vi "4channel.vi"() -> ()   [LabVIEW 2014]
doc: "Personal Daq 54 example.\nTriggering is immediate and readings are returned 1 scan at a time as available.\nBe sure to use the Acquisition Stop control for proper shutdown."
uses:
  <vilib>/Utility/error.llb/DialogType.ctl
  <vilib>/DAQmx/read.llb/DAQmx Read (Analog 1D DBL NChan 1Samp).vi
  <vilib>/Analysis/2dsp.llb/Complex FFT.vi
  <vilib>/DAQmx/create/channels.llb/DAQmx Create Channel (AI-Voltage-Basic).vi
  <vilib>/DAQmx/configure/timing.llb/DAQmx Timing (Sample Clock).vi
  <vilib>/DAQmx/miscellaneous.llb/DAQmx Fill In Error Info.vi
  <vilib>/measure/madcrms.llb/Basic Averaged DC-RMS for 1 Chan.vi
  Instance           2 26Saved   noise_Nov07_2009_5 .vi
  Instance          18 26Saved   noise_Nov07_2009_5 .vi
  <vilib>/express/express analysis/Spectral/Block/exnSpectralBlock spectral measurements peak poly.vi
  <vilib>/express/express analysis/Spectral/Block/exnSpectralBlock spectral measurements peak DDT.vi
  Instance           1 26Saved   noise_Nov07_2009_5 .vi
  Instance           4 26Saved   noise_Nov07_2009_5 .vi
  <vilib>/express/express analysis/Spectral/XNode/ExpressSpectralMeasurementsBlockNode.xnode
  <vilib>/measure/NI_MAPro.lvlib
  <vilib>/Analysis/NI_AALPro.lvlib
panel:
  out "I/Q Signal 2":dynamicdata(graph)
  in  "Save Data":bool
  in  "Max. Heartrate":i32=90
  in  "Min. Heartrate":i32=50
  out "Heartrate":dbl
  out "max value 2":dbl
  in  "Max. Resp. Rate":i32=30
  in  "Min. Resp. Rate":i32=10
  out "Resp. Rate":dbl
  out "max value":dbl
  out "Record":dynamicdata(graph)
  in  "input terminal configuration":i32(ring)=10083 items=["default"=-1, "RSE"=10083, "NRSE"=10078, "Differential"=10106, "Pseudodifferential"=12529]
  out "error out":errorcluster
  in  "stop":bool
  in  "Maximum Value":dbl=5.0 format="%0.2f"
  in  "Minimum Value":dbl=-2.0 format="%0.2f"
  in  "Rate":dbl=20.0 caption="Sample Rate (Hz)" format="%0.2f"
  in  "Samples per Channel":i32=1
  out "Combined Spectrum":waveform(dbl)(graph)
  out "I/Q Spectrum":dynamicdata(graph)
  out "Respiration Q":dbl=19.665142208058892 format="%#_3g"
  out "Respiration I":dbl=19.7 format="%#_3g"
  in  "FFT":i32=256
  out "I/Q Signal":dynamicdata(graph)
  in  "t0":timestamp=timestamp(3198752888.296 s since 1904-01-01)
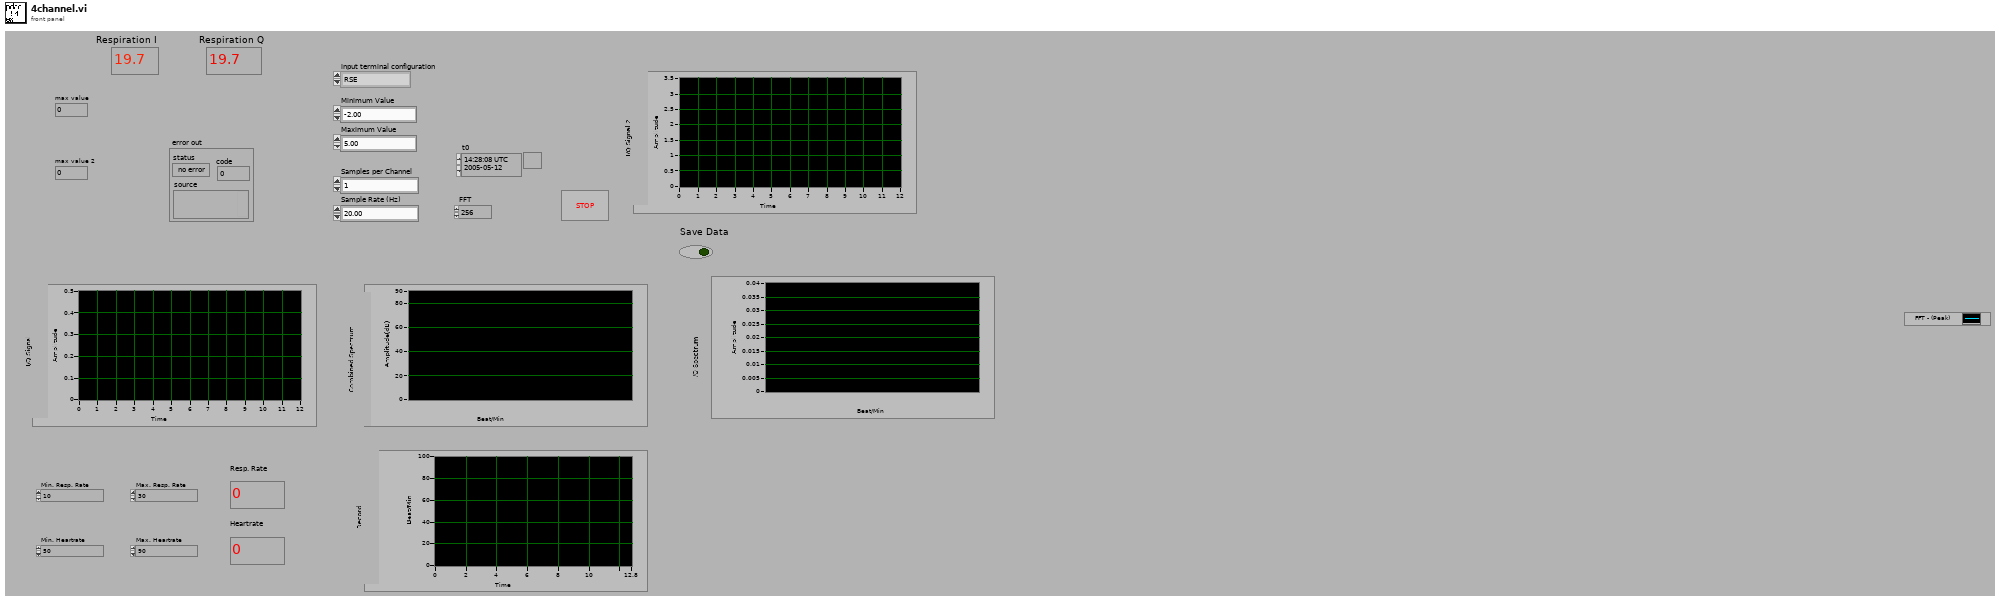
[diagram p1: front panel]
types:
  T1 = typedef "DialogType.ctl" = u16
  T2 = cluster{"averaging mode":u16, "weighting mode":u16, "number of averages":u32}
  T3 = cluster{"dB On (F)":bool, "unwrap phase (F)":bool, "convert to degree (F)":bool}
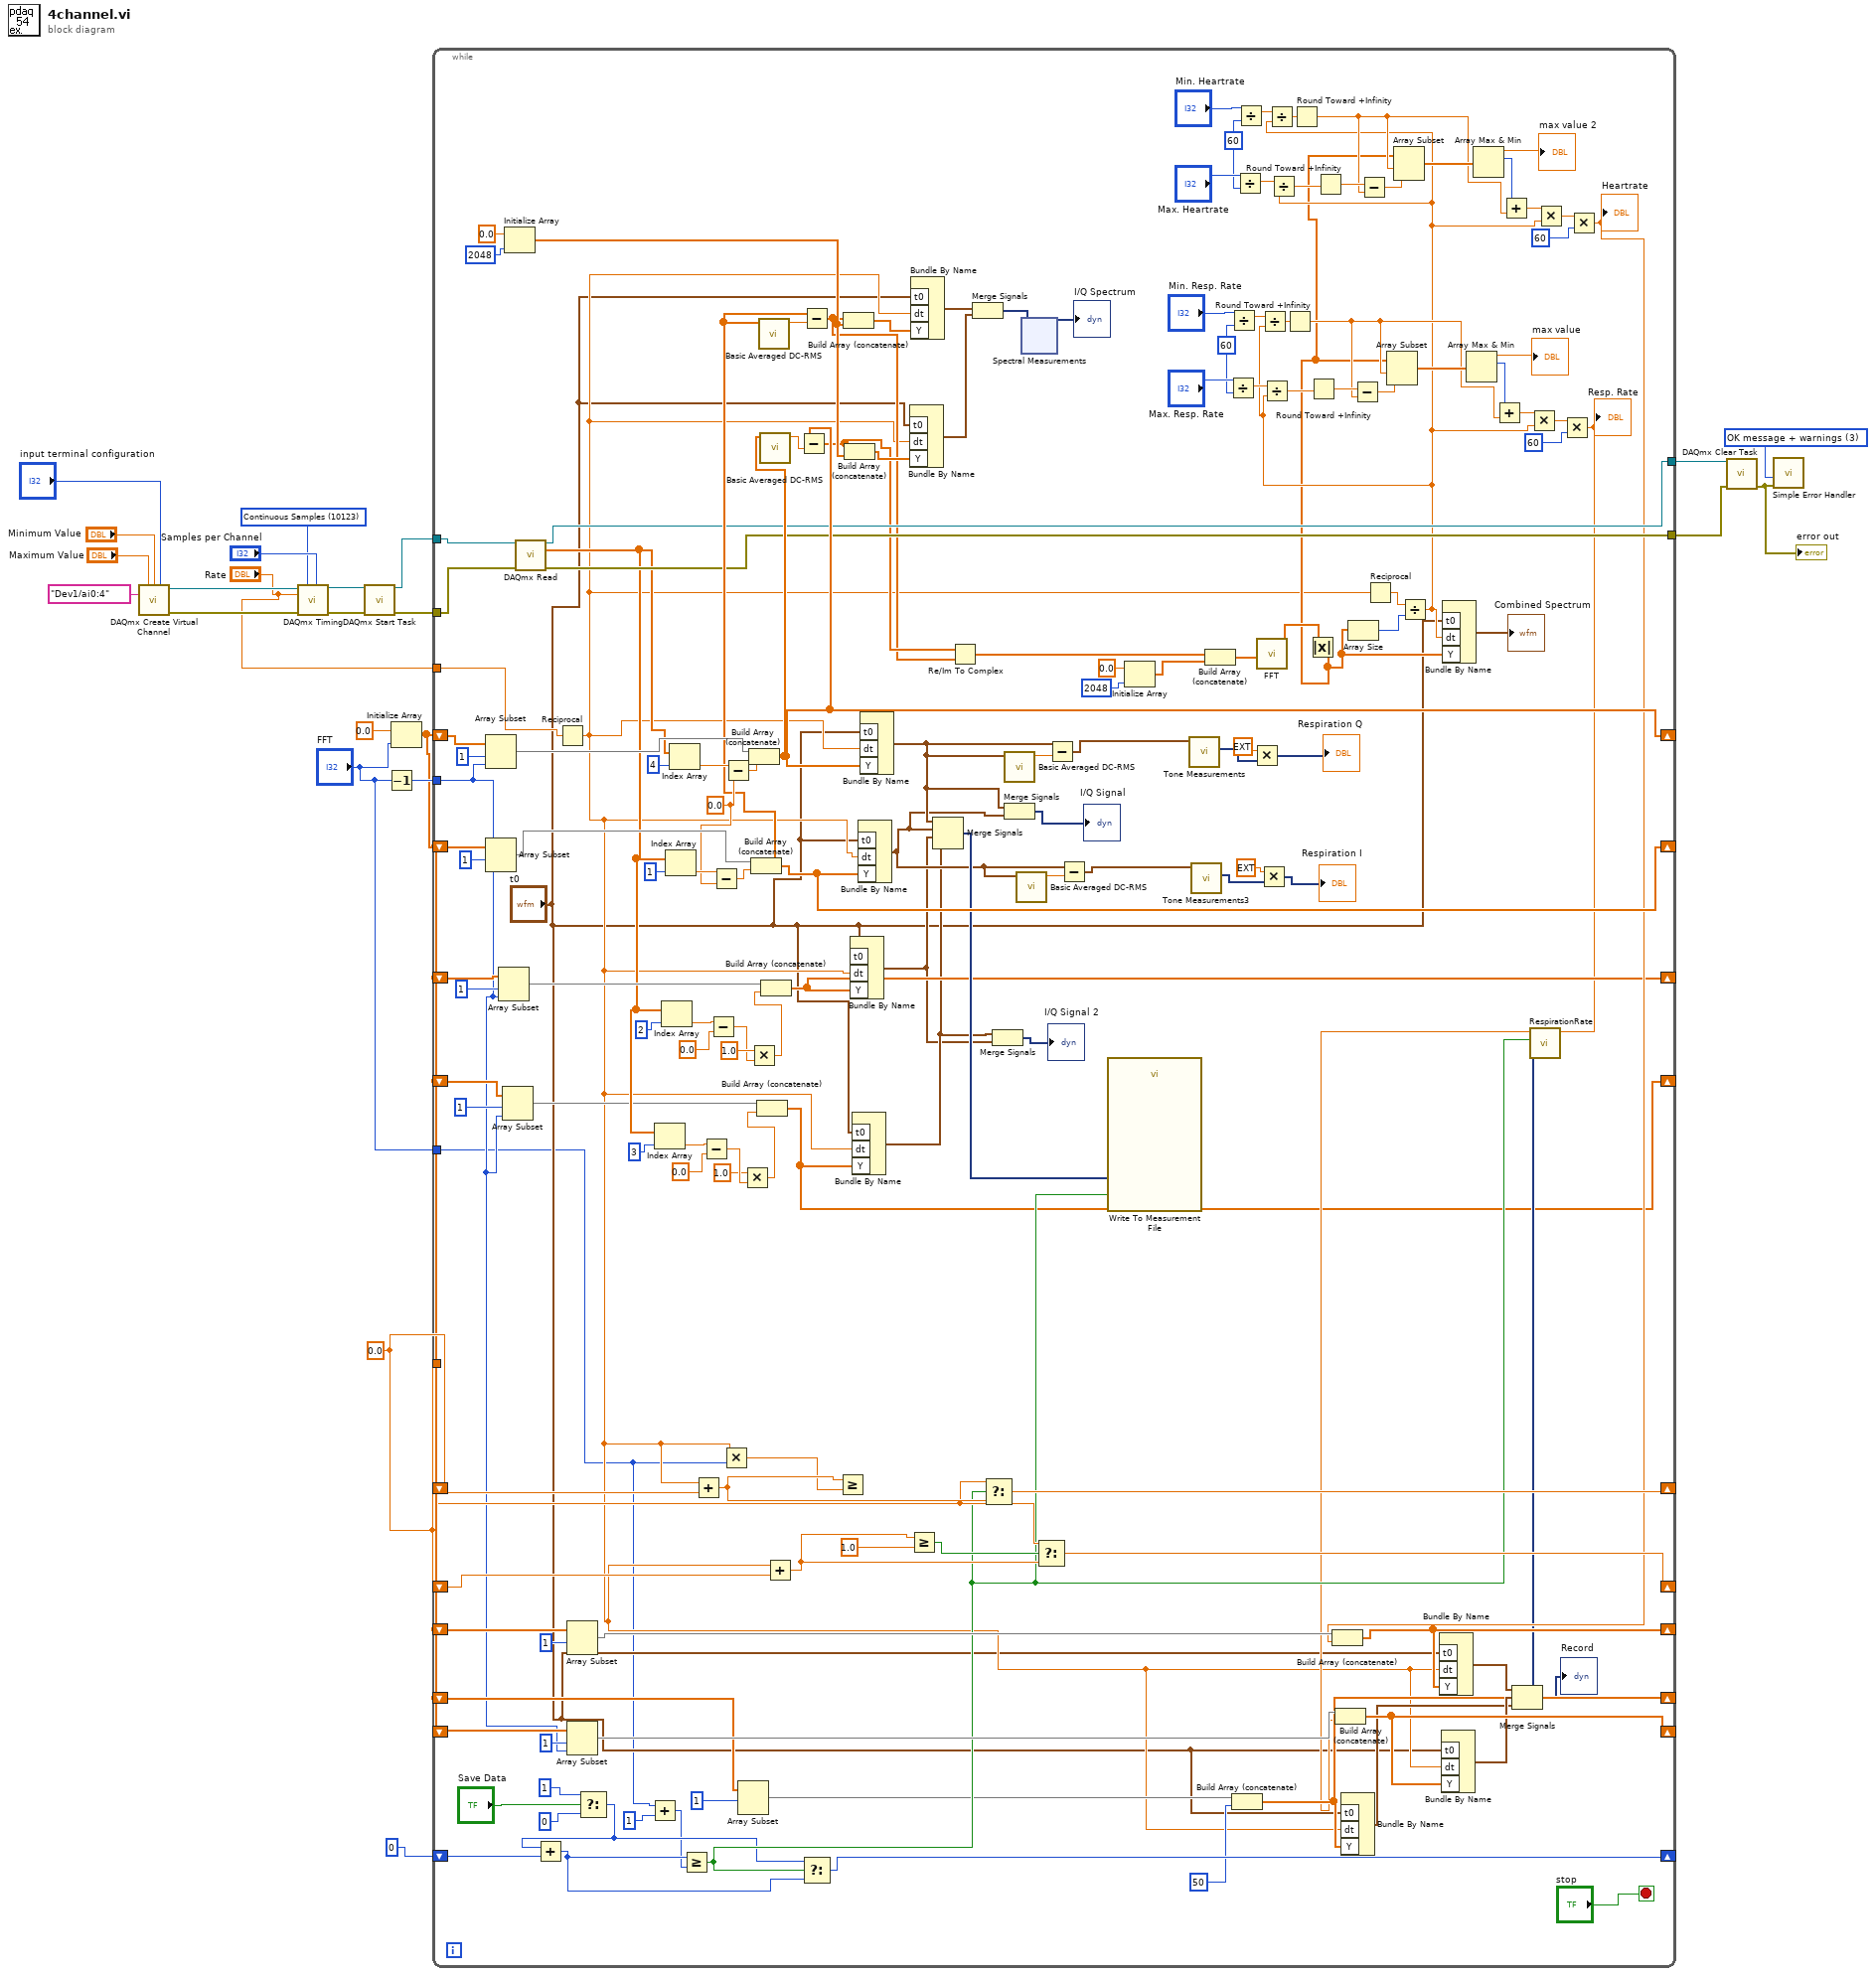
[diagram p0: block diagram]
diagram:
  w3 = 0.0 ("element")
  w9 = T1 3 items=["no dialog", "OK message", "continue or stop message", "OK message + warnings", "continue/stop + warnings"] ("type of dialog (OK msg:1)")
  w16 = 10123 items=["Finite Samples"=10178, "Continuous Samples"=10123] ("sample mode")
  n1 = call-poly <vilib>:"DAQmx Create Virtual Channel.vi"("maximum value"="Maximum Value", "minimum value"="Minimum Value", "input terminal configuration"="input terminal configuration", "physical channels"=tag "Dev1/ai0:4") -> ("task out"=w17:refnum<k21>, "error out"=w19:errorcluster)  [unwired: 5 in, 5 out]
  n2 = call-poly <vilib>:"DAQmx Timing.vi"("task/channels in"=w17, "sample mode"=w16, "samples per channel"="Samples per Channel", "rate"="Rate", "error in"=w19) -> ("task out"=w15:refnum<k21>, "error out"=w14:errorcluster)  [unwired: 2 in, 7 out]
  n3 = call <vilib>:"DAQmx Start Task.vi"("task/channels in"=w15, "error in"=w14) -> ("task out"=w12:refnum<k21>, "error out"=w11:errorcluster)  [unwired: 12 out]
  n4 = Decrement(x="FFT") -> (x-1=w22:i32)
  n5 = Initialize Array(0.0 ("element"), "FFT") -> (w1:dbl[])
  n6 = while {
    shift-right: [w148] -> _
    shift-left: w1 -> [w180]
    tunnel: w22 -> [w44]
    shift-right: [w147] -> _
    shift-left: w1 -> [w171]
    tunnel: w12 -> [w146]
    tunnel: w11 -> [w145]
    tunnel: "Rate" -> [w144]
    tunnel: [w143] -> w8
    tunnel: [w142] -> w7
    shift-right: [w134] -> _
    shift-left: w3 -> [w132]
    tunnel: "FFT" -> [w25]
    tunnel: w3 -> [w126]
    shift-right: [w130] -> _
    shift-left: w3 -> [w127]
    shift-right: [w112] -> _
    shift-left: w1 -> [w120]
    shift-right: [w113] -> _
    shift-left: w1 -> [w116]
    shift-right: [w71] -> _
    shift-left: 0 -> [w73]
    shift-right: [w58] -> _
    shift-left: w1 -> [w64]
    shift-right: [w53] -> _
    shift-left: w1 -> [w57]
    shift-right: [w33] -> _
    shift-left: w1 -> [w46]
    stop <- "stop" stop-if-true
    w76 = 60
    w92 = 60
    w165 = 0.0 ("element")
    n7 = Array Subset(array=w180, index=1, length=w44) -> (w178:dbl[])
    n8 = Array Subset(array=w171, index=1, length=w44) -> (w169:dbl[])
    n9 = Array Subset(array=w64, index=1, length=w44) -> (w59:dbl[])
    n10 = Array Subset(array=w46, index=1, length=w44) -> (w36:dbl[])
    n11 = Initialize Array(0.0 ("element"), 2048 ("dimension size")) -> (w139:dbl[])
    n12 = call-poly <vilib>:"DAQmx Read.vi"("task/channels in"=w146, "error in"=w145) -> ("task out"=w143:refnum<k21>, "data"=w37:dbl[], "error out"=w142:errorcluster)  [unwired: 11 out]
    n13 = Reciprocal(x=w144) -> (1/x=w35:dbl)
    n14 = Array Subset(array=w116, index=1) -> (w115:dbl[])  [unwired: 1 in]
    n15 = Array Subset(array=w120, index=1, length=w44) -> (w119:dbl[])
    n16 = Select(t=1, s="Save Data", f=0) -> (s? t:f=w67:i32)
    n17 = Add(x=w67, y=w73) -> (x+y=w72:i32)
    n18 = Add(x=w25, y=1 ("index")) -> (x+y=w24:i32)
    n19 = Index Array(array=w37, index=3 ("index (row)")) -> (element=w40:dbl)
    n20 = Index Array(array=w37, index=2 ("index (row)")) -> (element=w61:dbl)
    n21 = Index Array(array=w37, index=1 ("index (row)")) -> (element=w166:dbl)
    n22 = Index Array(array=w37, index=4 ("index (row)")) -> (element=w167:dbl)
    n23 = Greater Or Equal?(x=w72, y=w24) -> (x >= y?=w70:bool)
    n24 = Add(x=w35, y=w132) -> (x+y=w135:dbl)
    n25 = Subtract(x=w40, y=0.0 ("element")) -> (x-y=w43:dbl)
    n26 = Subtract(x=w61, y=0.0 ("element")) -> (x-y=w48:dbl)
    n27 = Subtract(x=w166, y=w165) -> (x-y=w158:dbl)
    n28 = Multiply(x=w35, y=w25) -> (x*y=w133:dbl)
    n29 = Subtract(x=w167, y=w165) -> (x-y=w159:dbl)
    n30 = Array Subset(array=w57, index=1) -> (w55:dbl[])  [unwired: 1 in]
    n31 = Multiply(x=1.0, y=w43) -> (x*y=w38:dbl)
    n32 = Build Array (concatenate)(w178, w159) -> (w148:dbl[])
    n33 = Multiply(x=1.0, y=w48) -> (x*y=w47:dbl)
    n34 = Build Array (concatenate)(w169, w158) -> (w147:dbl[])
    n35 = Build Array (concatenate)(w36, w38) -> (w33:dbl[])
    n36 = call-poly <vilib>:"Basic Averaged DC-RMS.vi"("signal in"=w147) -> ("DC value"=w157:dbl)  [unwired: 4 in, 6 out]
    n37 = call-poly <vilib>:"Basic Averaged DC-RMS.vi"("signal in"=w148) -> ("DC value"=w156:dbl)  [unwired: 4 in, 6 out]
    n38 = Build Array (concatenate)(w59, w47) -> (w58:dbl[])
    n39 = Add(x=w35, y=w127) -> (x+y=w131:dbl)
    n40 = Subtract(x=w148, y=w156) -> (x-y=w137:dbl[])
    n41 = Subtract(x=w147, y=w157) -> (x-y=w136:dbl[])
    n42 = Select(t=w67, s=w70, f=w72) -> (s? t:f=w71:i32)
    n43 = Greater Or Equal?(x=w135, y=w133) -> ()  [unwired: 1 out]
    n44 = Build Array (concatenate)(w136, w139) -> (w163:dbl[])
    n45 = Build Array (concatenate)(w137, w139) -> (w164:dbl[])
    n46 = Bundle By Name("t0"="t0", "dt"=w35, "Y"=w58) -> (w28:waveform(dbl))  [unwired: 1 out]
    n47 = Bundle By Name("t0"="t0", "dt"=w35, "Y"=w33) -> (w29:waveform(dbl))  [unwired: 1 out]
    n48 = Bundle By Name("t0"="t0", "dt"=w35, "Y"=w147) -> (w31:waveform(dbl))  [unwired: 1 out]
    n49 = Bundle By Name("t0"="t0", "dt"=w35, "Y"=w148) -> (w32:waveform(dbl))  [unwired: 1 out]
    n50 = Greater Or Equal?(x=w131, y=1.0) -> (x >= y?=w128:bool)
    n51 = Bundle By Name("t0"="t0", "dt"=w35, "Y"=w164) -> (w153:waveform(dbl))  [unwired: 1 out]
    n52 = Bundle By Name("t0"="t0", "dt"=w35, "Y"=w163) -> (w154:waveform(dbl))  [unwired: 1 out]
    n53 = Merge Signals(w32, w31, w28, w29) -> (w138:dynamicdata)
    n54 = Re/Im To Complex(1:w136, 2:w137) -> (0:w160:cdb[])
    n55 = Merge Signals(w154, w153) -> (w155:dynamicdata)
    n56 = Select(t=w126, s=w70, f=w135) -> (s? t:f=w134:dbl)
    n57 = Merge Signals(w29, w28) -> (→"I/Q Signal 2":dynamicdata)
    n58 = call-poly <vilib>:"Basic Averaged DC-RMS.vi"("signal in"=w32) -> ("DC value"=w125:dbl)  [unwired: 4 in, 6 out]
    n59 = Merge Signals(w32, w31) -> (→"I/Q Signal":dynamicdata)
    n60 = call-poly <vilib>:"Basic Averaged DC-RMS.vi"("signal in"=w31) -> ("DC value"=w123:dbl)  [unwired: 4 in, 6 out]
    n61 = xnode "Spectral Measurements"("Signals"=w155) -> ("FFT - (Peak)"=→"I/Q Spectrum":dynamicdata)  [unwired: 2 in, 3 out]
    n62 = Select(t=w126, s=w128, f=w131) -> (s? t:f=w130:dbl)
    n63 = Subtract(x=w32, y=w125) -> (x-y=w124:waveform(dbl))
    n64 = Subtract(x=w31, y=w123) -> (x-y=w122:waveform(dbl))
    n65 = call "Write To Measurement File"("Signals"=w138, "Enable"=w70) -> ()  [unwired: 5 in, 13 out]
    n66 = Initialize Array(0.0 ("element"), 2048 ("dimension size")) -> (w161:dbl[])
    n67 = call "Tone Measurements"("Signals"=w124) -> ("Frequency"=w175:dynamicdata)  [unwired: 1 in, 9 out]
    n68 = call "Tone Measurements3"("Signals"=w122) -> ("Frequency"=w172:dynamicdata)  [unwired: 1 in, 9 out]
    n69 = Build Array (concatenate)(w160, w161) -> (w149:cdb[])
    n70 = Divide(x="Max. Resp. Rate", y=w92) -> (x/y=w107:dbl)
    n71 = Divide(x="Min. Resp. Rate", y=w92) -> (x/y=w108:dbl)
    n72 = Build Array (concatenate)(w55, 50 ("index")) -> (w53:dbl[])
    n73 = Divide(x="Max. Heartrate", y=w76) -> (x/y=w90:dbl)
    n74 = Divide(x="Min. Heartrate", y=w76) -> (x/y=w91:dbl)
    n75 = Multiply(x=ext 60.0, y=w175) -> (x*y=→"Respiration Q":dynamicdata)
    n76 = call-poly <vilib>:"FFT.vi"("X"=w149) -> ("FFT {X}"=w152:cdb[])  [unwired: 2 in, 8 out]
    n77 = Multiply(x=ext 60.0, y=w172) -> (x*y=→"Respiration I":dynamicdata)
    n78 = Absolute Value(x=w152) -> (abs(x)=w65:dbl[])
    n79 = Bundle By Name("t0"="t0", "dt"=w35, "Y"=w53) -> (w54:waveform(dbl))  [unwired: 1 out]
    n80 = Array Size(array=w65) -> (size(s)=w150:i32)
    n81 = Reciprocal(x=w35) -> (1/x=w95:dbl)
    n82 = Divide(x=w95, y=w150) -> (x/y=w75:dbl)
    n83 = Divide(x=w108, y=w75) -> (x/y=w106:dbl)
    n84 = Divide(x=w107, y=w75) -> (x/y=w105:dbl)
    n85 = Divide(x=w91, y=w75) -> (x/y=w89:dbl)
    n86 = Divide(x=w90, y=w75) -> (x/y=w88:dbl)
    n87 = Round Toward +Infinity(x=w106) -> (ceil(x): smallest int >= x=w99:dbl)
    n88 = Round Toward +Infinity(x=w89) -> (ceil(x): smallest int >= x=w82:dbl)
    n89 = Round Toward +Infinity(x=w105) -> (ceil(x): smallest int >= x=w103:dbl)
    n90 = Round Toward +Infinity(x=w88) -> (ceil(x): smallest int >= x=w86:dbl)
    n91 = Subtract(x=w103, y=w99) -> (x-y=w104:dbl)
    n92 = Subtract(x=w86, y=w82) -> (x-y=w87:dbl)
    n93 = Array Subset(array=w65, index=w99, length=w104) -> (w102:dbl[])
    n94 = Array Subset(array=w65, index=w82, length=w87) -> (w85:dbl[])
    n95 = Bundle By Name("t0"="t0", "dt"=w75, "Y"=w65) -> (→"Combined Spectrum":waveform(dbl))  [unwired: 1 out]
    n96 = Array Max & Min(array=w102) -> (max value=→"max value":dbl, max index (indices)=w100:i32)  [unwired: 2 out]
    n97 = Array Max & Min(array=w85) -> (max value=→"max value 2":dbl, max index (indices)=w83:i32)  [unwired: 2 out]
    n98 = Add(x=w100, y=w99) -> (x+y=w98:dbl)
    n99 = Add(x=w83, y=w82) -> (x+y=w81:dbl)
    n100 = Multiply(x=w98, y=w75) -> (x*y=w97:dbl)
    n101 = Multiply(x=w81, y=w75) -> (x*y=w80:dbl)
    n102 = Multiply(x=w97, y=60) -> (x*y=w51:dbl)
    "Resp. Rate" <- w51
    n103 = Build Array (concatenate)(w119, w51) -> (w112:dbl[])
    n104 = Bundle By Name("t0"="t0", "dt"=w35, "Y"=w112) -> (w110:waveform(dbl))  [unwired: 1 out]
    n105 = Multiply(x=w80, y=60) -> (x*y=w74:dbl)
    "Heartrate" <- w74
    n106 = Build Array (concatenate)(w115, w74) -> (w113:dbl[])
    n107 = Bundle By Name("t0"="t0", "dt"=w35, "Y"=w113) -> (w111:waveform(dbl))  [unwired: 1 out]
    n108 = Merge Signals(w111, w110, w54) -> (w52:dynamicdata)
    "Record" <- w52
    n109 = call "RespirationRate"("Enable"=w70, "Signals"=w52) -> ()  [unwired: 3 in, 7 out]
  }
  n110 = call <vilib>:"DAQmx Clear Task.vi"("task in"=w8, "error in"=w7) -> ("error out"=w6:errorcluster)  [unwired: 13 out]
  "error out" <- w6
  n111 = call <vilib>:"Simple Error Handler.vi"("type of dialog (OK msg:1)"=w9, "error in (no error)"=w6) -> ()  [unwired: 8 out]
